vi "Picture_Square_ROI.vi"(10 "Square":bool, 11 "Cluster":T2) -> (3 "Cluster 2":T1)   [LabVIEW 2009]
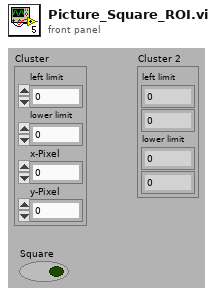
[diagram p1: front panel]
types:
  T1 = cluster{"left limit":i32, i32, "lower limit":i32, i32}
  T2 = cluster{"left limit":i32, "lower limit":i32, "x-Pixel":i32, "y-Pixel":i32}
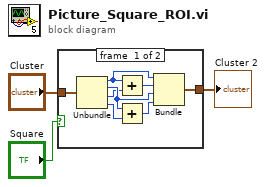
[diagram p0: block diagram]
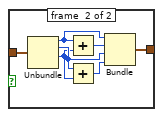
[diagram p2: hidden frame]
diagram:
  n1 = case shown="False" "Square" {
    tunnel: "Cluster" -> [w11 w15]
    tunnel: [w9 w18] -> w1
    frame #0 {
      n2 = Unbundle(w11) -> ("left limit"=w8:i32, "lower limit"=w6:i32, "x-Pixel"=w4:i32, "y-Pixel"=w10:i32)
      n3 = Add(x=w8, y=w4) -> (x+y=w7:i32)
      n4 = Add(x=w6, y=w10) -> (x+y=w5:i32)
      n5 = Bundle("left limit"=w8, w7, "lower limit"=w6, w5) -> (w9:T1)  [unwired: 1 out]
    }
    frame #1 {
      n6 = Unbundle(w15) -> ("left limit"=w14:i32, "lower limit"=w13:i32, "x-Pixel"=w12:i32)  [unwired: 1 out]
      n7 = Add(x=w14, y=w12) -> (x+y=w17:i32)
      n8 = Add(x=w13, y=w12) -> (x+y=w16:i32)
      n9 = Bundle("left limit"=w14, w17, "lower limit"=w13, w16) -> (w18:T1)  [unwired: 1 out]
    }
  }
  "Cluster 2" <- w1
